vi "Overhaul.vi"(9 "goal node reference":refnum<data-value>, 10 "start node reference":refnum<data-value>, 11 "RVCLibrary_Bug2 in":refnum<class "RVCLibrary_Bug2.lvclass">) -> (3 "RVCLibrary_Bug2 out":refnum<class "RVCLibrary_Bug2.lvclass">)   [LabVIEW 2013, in "RVCLibrary_Bug2.lvclass"]
uses:
  RVCLibrary_Bug2.lvclass
  <vilib>/robotics/Navigation/shared/MapNode/AbstractDstarNode/NI_Robotics_AbstractDstarNode.lvclass
  RVCLibrary_Bug2.lvclass/RVCLibrary_Bug2.ctl
  <vilib>/robotics/Navigation/shared/Priority Queue/NI_Robotics_Priority Queue.lvclass
  <vilib>/robotics/Navigation/shared/InconsistentList/NI_Robotics_InconsistentList.lvclass
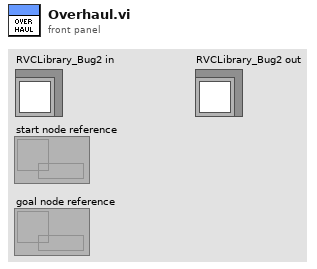
[diagram p1: front panel]
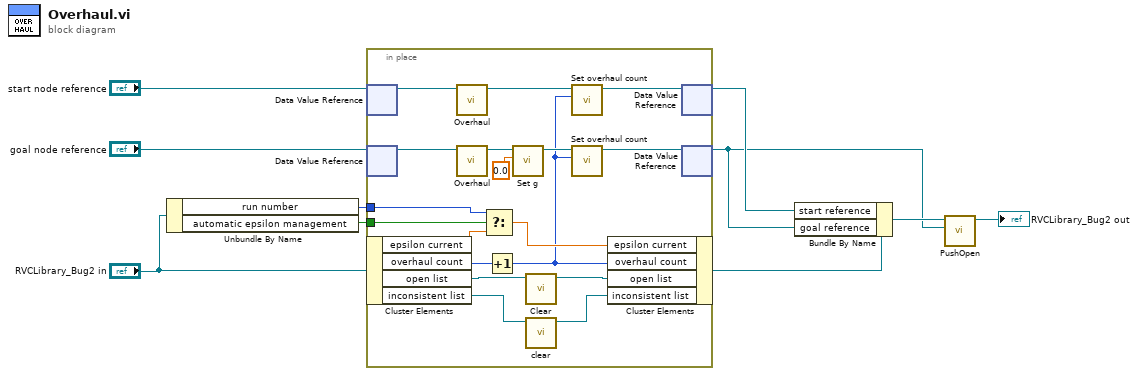
[diagram p0: block diagram]
diagram:
  n1 = Unbundle By Name("RVCLibrary_Bug2 in") -> ("run number"=w7:i32, "automatic epsilon management"=w8:bool)
  n2 = in-place {
    in-place-border: w8 -> [w23]
    in-place-border: w7 -> [w22]
    n3 = in-place-dvr #1("start node reference") -> (w18:refnum<class "NI_Robotics_AbstractDstarNode.lvclass">)  [unwired: 1 out]
    n4 = in-place-dvr #2("goal node reference") -> (w13:refnum<class "NI_Robotics_AbstractDstarNode.lvclass">)  [unwired: 1 out]
    n5 = in-place-cluster #3("RVCLibrary_Bug2 in") -> ("epsilon current"=w20:dbl, "overhaul count"=w28:i32, "open list"=w27:refnum<class "NI_Robotics_Priority Queue.lvclass">, "inconsistent list"=w25:refnum<class "NI_Robotics_InconsistentList.lvclass">)
    n6 = call <vilib>:"Overhaul.vi"("AbstractDstarNode in"=w18) -> ("AbstractDstarNode out"=w19:refnum<class "NI_Robotics_AbstractDstarNode.lvclass">)  [unwired: 10 in]
    n7 = call <vilib>:"Overhaul.vi"("AbstractDstarNode in"=w13) -> ("AbstractDstarNode out"=w15:refnum<class "NI_Robotics_AbstractDstarNode.lvclass">)  [unwired: 10 in]
    n8 = Select(t=w22, s=w23, f=w20) -> (s? t:f=w21:dbl)
    n9 = Increment(x=w28) -> (x+1=w11:i32)
    n10 = call <vilib>:"Set g.vi"("g"=0.0, "AbstractDstarNode in"=w15) -> ("AbstractDstarNode out"=w16:refnum<class "NI_Robotics_AbstractDstarNode.lvclass">)  [unwired: 9 in]
    n11 = call <vilib>:"Clear.vi"("Priority Queue in"=w27) -> ("Priority Queue out"=w26:refnum<class "NI_Robotics_Priority Queue.lvclass">)  [unwired: 8 in, 2 out]
    n12 = call <vilib>:"clear.vi"("InconsistentList in"=w25) -> ("InconsistentList out"=w24:refnum<class "NI_Robotics_InconsistentList.lvclass">)  [unwired: 9 in, 1 out]
    n13 = call <vilib>:"Set overhaul count.vi"("overhaul count"=w11, "AbstractDstarNode in"=w19) -> ("AbstractDstarNode out"=w17:refnum<class "NI_Robotics_AbstractDstarNode.lvclass">)  [unwired: 9 in]
    n14 = call <vilib>:"Set overhaul count.vi"("overhaul count"=w11, "AbstractDstarNode in"=w16) -> ("AbstractDstarNode out"=w12:refnum<class "NI_Robotics_AbstractDstarNode.lvclass">)  [unwired: 9 in]
    n15 = in-place-cluster #3("epsilon current"=w21, "overhaul count"=w11, "open list"=w26, "inconsistent list"=w24) -> (w10:refnum<class "RVCLibrary_Bug2.lvclass">)
    n16 = in-place-dvr #1(w17) -> (w5:refnum<data-value>)  [unwired: 1 out]
    n17 = in-place-dvr #2(w12) -> (w3:refnum<data-value>)  [unwired: 1 out]
  }
  n18 = Bundle By Name(cluster=w10, "start reference"=w5, "goal reference"=w3) -> (w9:refnum<class "RVCLibrary_Bug2.lvclass">)
  n19 = call "PushOpen.vi"("node ref in"=w3, "RVCLibrary_Bug in"=w9) -> ("RVCLibrary_Bug out"=→"RVCLibrary_Bug2 out":refnum<class "RVCLibrary_Bug2.lvclass">)  [unwired: 8 in, 1 out]
